vi "modulo.vi"(11 "X1":dbl) -> (3 "Result":dbl)   [LabVIEW 2020]
panel:
  out "Quotient & Remainder":dbl
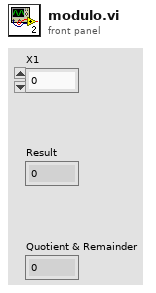
[diagram p1: front panel]
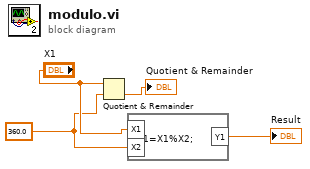
[diagram p0: block diagram]
diagram:
  w1 = 360.0 ("X2")
  n1 = Quotient & Remainder(x="X1", y=w1) -> (floor(x/y)=→"Quotient & Remainder":dbl)  [unwired: 1 out]
  n2 = formula code="Y1=X1%X2;"("X1"="X1", "X2"=w1) -> ("Y1"=→"Result":dbl)
